vi "GE 5565PIORC.Memory.VISA Move In-Place (DBL).vi"(5 "count (-1: all)":i32=-1, 7 "address space":T1=1 items=["VXI/VME A16"=1, "VXI/VME A24"=2, "VXI/VME A32"=3, "VXI/VME A64"=4, "PXI Memory Allocations"=9, "PXI Configuration"=10, "PXI BAR0"=11, "PXI BAR1"=12, "PXI BAR2"=13, "PXI BAR3"=14, "PXI BAR4"=15, "PXI BAR5"=16], 8 "error in (no error)":errorcluster, 9 "data in":dbl[](array[numeric]), 10 "offset (0)":u32, 11 "VISA resource name":refnum<visa-resource-name>) -> (0 "error out":errorcluster, 1 "data out":dbl[](array[numeric]), 3 "VISA resource name out":refnum<visa-resource-name>)   [LabVIEW 2016, in "GE 5565PIORC.lvclass"]
uses:
  GE 5565PIORC.lvclass
  <vilib>/Instr/_visa.llb/VISA Register Access Address Space.ctl
  visa32.dll
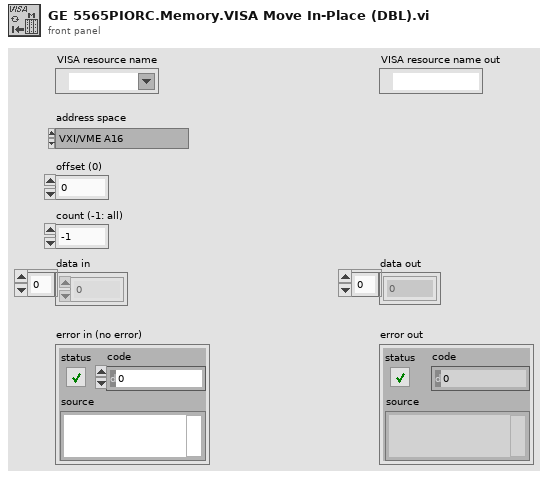
[diagram p1: front panel]
types:
  T1 = typedef "VISA Register Access Address Space.ctl" = u16
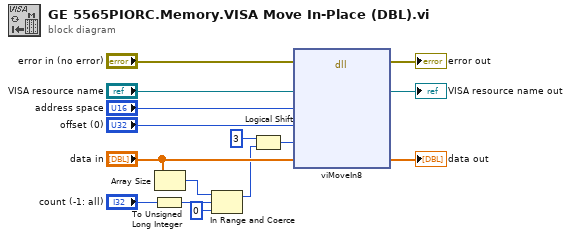
[diagram p0: block diagram]
diagram:
  n1 = To Unsigned Long Integer(number="count (-1: all)") -> (unsigned 32bit integer=w2:u32)
  n2 = Array Size(array="data in") -> (size(s)=w5:i32)
  n3 = In Range and Coerce(upper limit=w5, x=w2, lower limit=u32 0) -> (coerced(x)=w3:u32)  [unwired: 1 out]
  n4 = Logical Shift(y=i16 3, x=w3) -> (x << y=w8:u32)
  n5 = dll-call lib="visa32.*" fn="viMoveIn8"(error in="error in (no error)", "session"="VISA resource name", "address space"="address space", "offset"="offset (0)", "size"=w8, "data"="data in") -> (error out=→"error out":errorcluster, "session"=→"VISA resource name out":refnum<visa-resource-name>, "data"=→"data out":dbl[])  [unwired: 6 in, 1 out]
